vi "Teleop.vi"() -> ()   [LabVIEW 2017]
doc: "This VI is called for each TeleOp packet received from the DS where the robot is not disabled. It is often used to read from the joysticks and update I/O or to update setpoints for timed control loops. It should complete and return within 20 milliseconds or it may miss DS packets."
uses:
  <vilib>/Rock Robotics/WPI/DriverStation/WPI_DriverStationDerivedRobotMode.ctl
  <vilib>/Rock Robotics/WPI/DriverStation/WPI_DriverStationRobotMode2.ctl
  <vilib>/Rock Robotics/WPI/DriverStation/WPI_DriverStationMatch Info.ctl
  <vilib>/Rock Robotics/WPI/Joystick/WPI_JoystickDeviceEnum.ctl
  <vilib>/Rock Robotics/SystemInterfaces/DIO/FPGA_DIOPWMChannel.ctl
  <vilib>/Rock Robotics/SystemInterfaces/DIO/FPGA_DIOChannel.ctl
  <vilib>/Rock Robotics/WPI/MotorControl/WPI_MotorControlOpen SPARK.vi
  <vilib>/Rock Robotics/WPI/Switch/WPI_SwitchOpenLimit.vi
  <vilib>/Rock Robotics/WPI/RobotDrive/WPI_RobotDriveOpen2MotorWithSPARK.vi
  <vilib>/Rock Robotics/WPI/RobotDrive/WPI_RobotDriveArcadeDrive_Standard(NoSaturation).vi
panel:
  in  "Match Info":T1={"Autonomous Elapsed Seconds"=0.0, "TeleOp Elapsed Seconds"=0.0, "Disabled Elapsed Seconds"=0.0, "Visited Autonomous"=FALSE, "Visited TeleOp"=FALSE, "Visited Disabled"=FALSE, "Autonomous Settings"={"Autonomous Style"=enum."Independent", "VI Refnum"=refnum}}
  in  "Robot Mode":T2
  in  "Call Context":T3
  out "Switch Pressed 2":bool
  out "Switch Pressed":bool
  in  "stop 2":bool
  in  "stop":bool
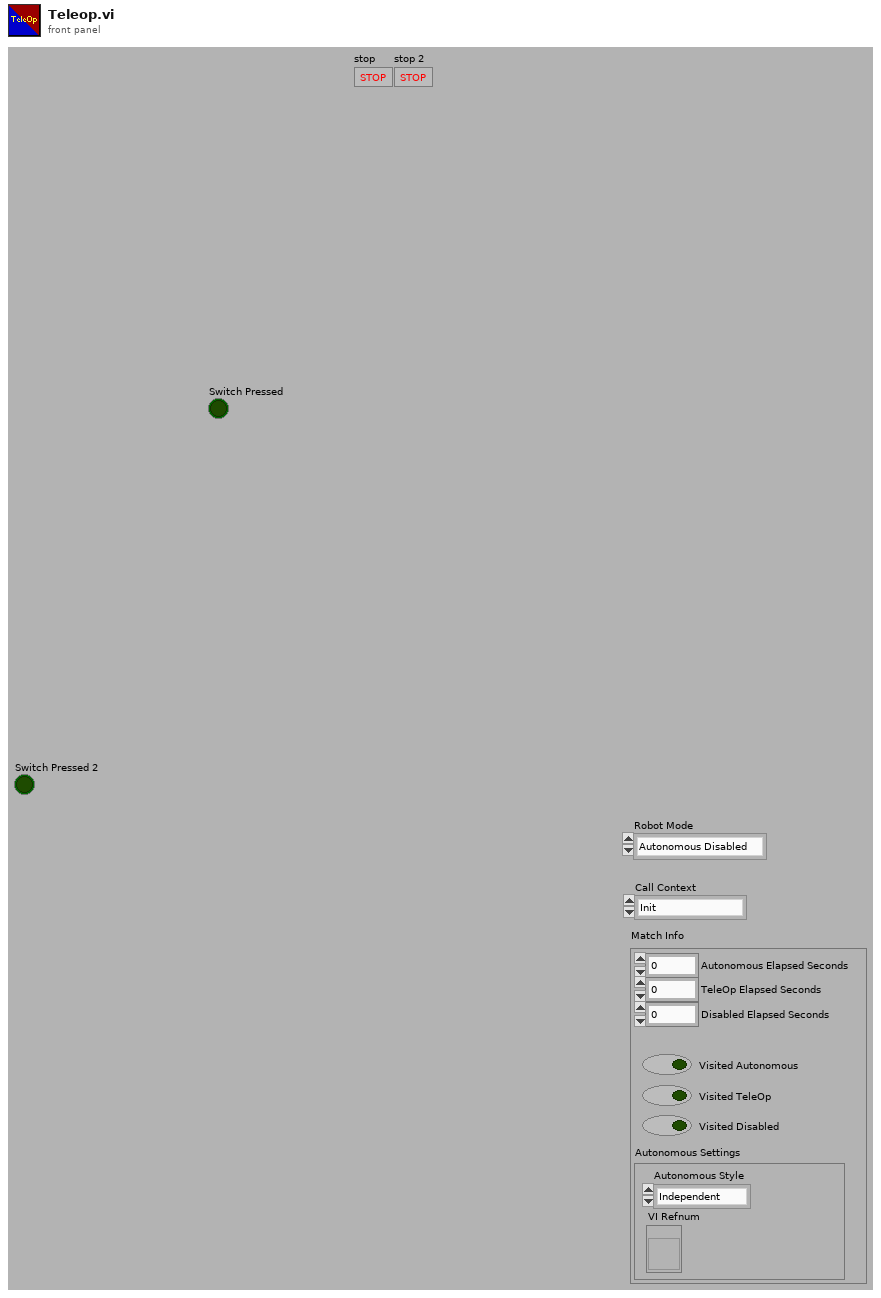
[diagram p1: front panel]
types:
  T1 = typedef "WPI_DriverStationMatch Info.ctl" = cluster{"Autonomous Elapsed Seconds":dbl, "TeleOp Elapsed Seconds":dbl, "Disabled Elapsed Seconds":dbl, "Visited Autonomous":bool, "Visited TeleOp":bool, "Visited Disabled":bool, "Autonomous Settings":cluster{"Autonomous Style":enum16{"Iterative", "Independent"}, "VI Refnum":refnum<vi>}}
  T2 = typedef "WPI_DriverStationRobotMode2.ctl" = enum16{"Autonomous Disabled", "Autonomous Enabled", "Teleop Disabled", "Teleop Enabled", "Disconnected", "Finish", "Test Disabled", "Test Enabled", "Emergency Stopped"}
  T3 = typedef "WPI_DriverStationDerivedRobotMode.ctl" = enum16{"Init", "Execute", "Stop"}
  T4 = typedef "FPGA_DIOPWMChannel.ctl" = enum8{"PWM 0", "PWM 1", "PWM 2", "PWM 3", "PWM 4", "PWM 5", "PWM 6", "PWM 7", "PWM 8", "PWM 9", "PWM MXP 0", "PWM MXP 1", "PWM MXP 2", "PWM MXP 3", "PWM MXP 4", "PWM MXP 5", "PWM MXP 6", "PWM MXP 7", "PWM MXP 8", "PWM MXP 9", "Invalid"}
  T5 = typedef "FPGA_DIOChannel.ctl" = enum8{"DIO 0", "DIO 1", "DIO 2", "DIO 3", "DIO 4", "DIO 5", "DIO 6", "DIO 7", "DIO 8", "DIO 9", "DIO MXP 0", "DIO MXP 1", "DIO MXP 2", "DIO MXP 3", "DIO MXP 4", "DIO MXP 5", "DIO MXP 6", "DIO MXP 7", "DIO MXP 8", "DIO MXP 9", "DIO MXP 10", "DIO MXP 11", "DIO MXP 12", "DIO MXP 13", "DIO MXP 14", "DIO MXP 15", "SPI Port CS1", "SPI Port CS2", "SPI Port CS3", "SPI Port MISO", "SPI Port MOSI", "Invalid"}
  T6 = typedef "WPI_JoystickDeviceEnum.ctl" = enum16{"USB 0", "USB 1", "USB 2", "USB 3", "USB 4", "USB 5"}
  T7 = typedef "WPI_MotorControlDeviceRef.ctl" = cluster{"DeviceStatus":errorcluster, "Type":T8, "PWM":cluster{"PWM Channel":T4, "DeadBand":T9}, "CAN":cluster{"Device Number":u8, "SetOutput VI Ref":variant, "GetOutput VI Ref":variant, "Enable VI Ref":variant, "Disable VI Ref":variant, "Data":variant}, "Invert":bool, "DIO PWM":cluster{"PWM \"Enable\" Channel":T4, "DIOChannel":T5, "PWM Rate":dbl}}
  T8 = typedef "WPI_MotorControlType.ctl" = enum16{"PWM", "CAN", "DIO PWM"}
  T9 = typedef "WPI_PWMDeadband.ctl" = cluster{"Name":string, "maxPositivePwm":i32, "minPositivePwm":i32, "centerPwm":i32, "maxNegativePwm":i32, "minNegativePwm":i32, "angularRange":u16}
  T10 = typedef "WPI_SwitchDevRef.ctl" = cluster{"DevStatus":errorcluster, "DIO Channel":T5, "CntIndex":T11, "Normally Closed":bool}
  T11 = typedef "FPGA_CounterCtrSystemIndex.ctl" = enum8{"Ctr 0", "Ctr 1", "Ctr 2", "Ctr 3", "Ctr 4", "Ctr 5", "Ctr 6", "Ctr 7", "Invalid"}
  T12 = typedef "WPI_JoystickDevRef.ctl" = cluster{"Device":T6}
  T13 = typedef "WPI_RobotDriveDevRef.ctl" = cluster{"DevStatus":errorcluster, "Motors[]":T7[], "Square Inputs":bool, "Max Output":dbl}
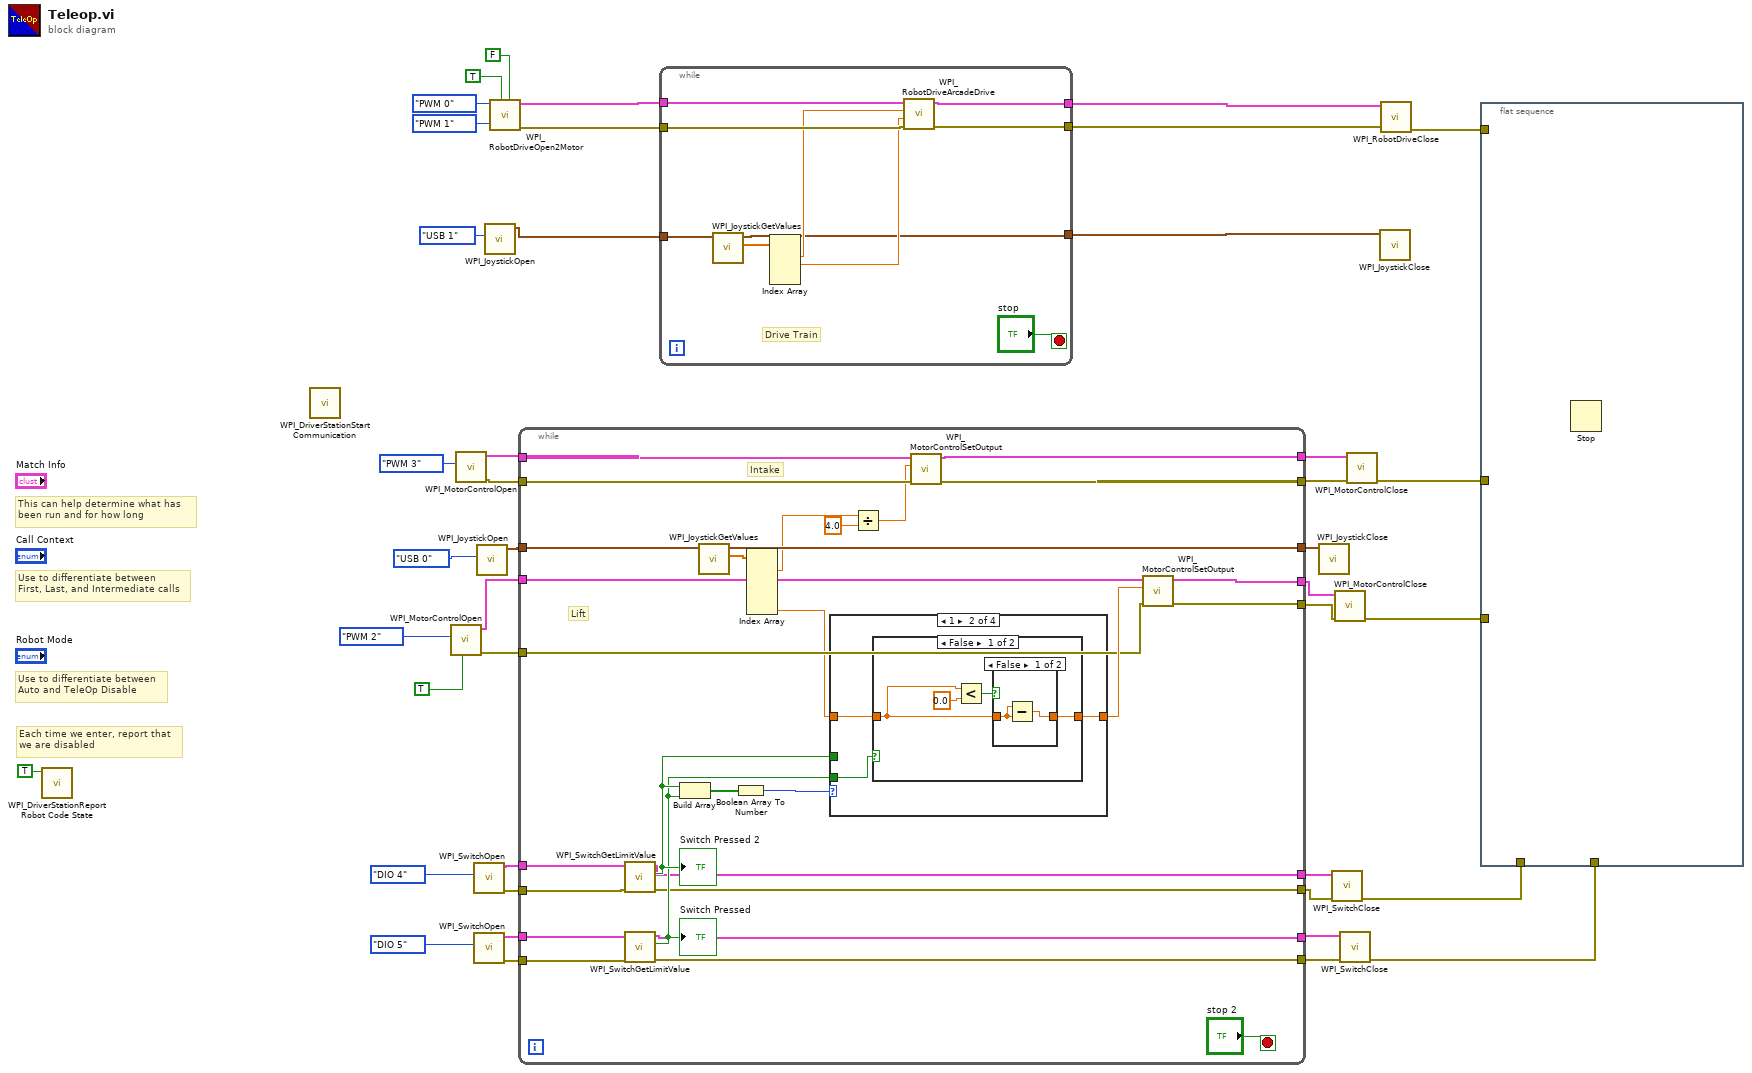
[diagram p0: block diagram]
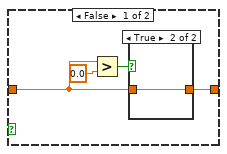
[diagram p6: hidden frame]
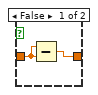
[diagram p7: hidden frame]
diagram:
  # "Each time we enter, report that\nwe are disabled"
  # "Use to differentiate between\nFirst, Last, and Intermediate calls"
  # "This can help determine what has\nbeen run and for how long"
  # "Use to differentiate between\nAuto and TeleOp Disable"
  n1 = call <vilib>:"WPI_DriverStationReport Robot Code State.vi"("Disabled"=TRUE ("Autonomous")) -> ()  [unwired: 10 in, 1 out]
  n2 = call <vilib>:"WPI_DriverStationStart Communication.vi"() -> ()  [unwired: 12 in]
  n3 = call-poly <vilib>:"WPI_MotorControlOpen.vi"("Invert"=TRUE, "PWM Channel"=FPGA_DIOPWMChannel."PWM 2" ("suck")) -> ("error out"=w15:errorcluster, "MotorControlDeviceRef"=w16:T7)  [unwired: 8 in]
  n4 = call-poly <vilib>:"WPI_MotorControlOpen.vi"("PWM Channel"=FPGA_DIOPWMChannel."PWM 3") -> ("error out"=w28:errorcluster, "MotorControlDeviceRef"=w31:T7)  [unwired: 9 in]
  n5 = call-poly <vilib>:"WPI_SwitchOpen.vi"("DIO Channel"=FPGA_DIOChannel."DIO 4") -> ("error out"=w19:errorcluster, "SwitchDevRef"=w20:T10)  [unwired: 9 in]
  n6 = call-poly <vilib>:"WPI_SwitchOpen.vi"("DIO Channel"=FPGA_DIOChannel."DIO 5") -> ("error out"=w17:errorcluster, "SwitchDevRef"=w18:T10)  [unwired: 9 in]
  n7 = call <vilib>:"WPI_JoystickOpen.vi"("JoystickDevice"=WPI_JoystickDeviceEnum."USB 0") -> ("JoystickDevRef"=w26:T12)  [unwired: 10 in]
  n8 = call <vilib>:"WPI_JoystickOpen.vi"("JoystickDevice"=WPI_JoystickDeviceEnum."USB 1") -> ("JoystickDevRef"=w41:T12)  [unwired: 10 in]
  n9 = call-poly <vilib>:"WPI_RobotDriveOpen2Motor.vi"("Right Motor Inverted"=FALSE, "Left Motor Inverted"=TRUE, "Right Motor"=FPGA_DIOPWMChannel."PWM 1", "Left Motor"=FPGA_DIOPWMChannel."PWM 0") -> ("error out"=w38:errorcluster, "RobotDriveDevRef"=w39:T13)  [unwired: 6 in]
  n10 = while {
    tunnel: w31 -> [w70]
    tunnel: [w69] -> w30
    tunnel: [w68] -> w29
    tunnel: w28 -> [w67]
    tunnel: w26 -> [w66]
    tunnel: [w64] -> w25
    tunnel: w20 -> [w58]
    tunnel: w19 -> [w57]
    tunnel: w18 -> [w56]
    tunnel: w17 -> [w55]
    tunnel: w16 -> [w54]
    tunnel: w15 -> [w53]
    tunnel: [w52] -> w9
    tunnel: [w51] -> w10
    tunnel: [w50] -> w14
    tunnel: [w49] -> w11
    tunnel: [w48] -> w12
    tunnel: [w47] -> w13
    stop <- "stop 2" stop-if-true
    # "Lift"
    # "Intake"
    n11 = call <vilib>:"WPI_SwitchGetLimitValue.vi"("error in (no error)"=w57, "SwitchDevRef"=w58) -> ("error out"=w49:errorcluster, "Switch Pressed"=w60:bool, "SwitchDevRef"=w50:T10)  [unwired: 7 in]
    "Switch Pressed 2" <- w60
    n12 = call <vilib>:"WPI_SwitchGetLimitValue.vi"("error in (no error)"=w55, "SwitchDevRef"=w56) -> ("error out"=w47:errorcluster, "Switch Pressed"=w59:bool, "SwitchDevRef"=w48:T10)  [unwired: 7 in]
    "Switch Pressed" <- w59
    n13 = Build Array(w60, w59) -> (w63:bool[])
    n14 = call <vilib>:"WPI_JoystickGetValues.vi"("JoystickDevRef"=w66) -> ("Axes"=w65:dbl[], "JoystickDevRef"=w64:T12)  [unwired: 6 in, 3 out]
    n15 = Boolean Array To Number(Boolean array=w63) -> (number=w62:u32)
    n16 = Index Array(array=w65) -> (element #1=w43:dbl, element #6=w42:dbl)  [unwired: 6 in, 4 out]
    n17 = case shown="1" w62 {
      tunnel: [w71 w74 w85 w94] -> w61
      tunnel: w59 -> [_ w73 _ _]
      tunnel: w60 -> [_ _ w84 _]
      tunnel: w42 -> [w71 w72 w83 w94]
      frame 0, Default {
      }
      frame 1 {
        n18 = case shown="False" w73 {
          tunnel: [w76 w82] -> w74
          tunnel: w72 -> [w75 w82]
          frame False {
            n19 = Less?(x=w75, y=0.0) -> (x < y?=w77:bool)
            n20 = case shown="False" w77 {
              tunnel: [w80 w81] -> w76
              tunnel: w75 -> [w79 w81]
              frame False {
                n21 = Subtract(x=w79, y=w79) -> (x-y=w80:dbl)
              }
              frame True {
              }
            }
          }
          frame True {
          }
        }
      }
      frame 2 {
        n22 = case shown="True" w84 {
          tunnel: [w87 w93] -> w85
          tunnel: w83 -> [w86 w93]
          frame False {
            n23 = Greater?(x=w86, y=0.0) -> (0:w88:bool)
            n24 = case shown="True" w88 {
              tunnel: [w91 w92] -> w87
              tunnel: w86 -> [w90 w92]
              frame False {
                n25 = Subtract(x=w90, y=w90) -> (x-y=w91:dbl)
              }
              frame True {
              }
            }
          }
          frame True {
          }
        }
      }
      frame 3 {
      }
    }
    n26 = Divide(x=w43, y=4.0) -> (x/y=w45:dbl)
    n27 = call <vilib>:"WPI_MotorControlSetOutput.vi"("error in (no error)"=w67, "Output"=w45, "MotorControlDevRef"=w70) -> ("error out"=w68:errorcluster, "MotorControlDevRef"=w69:T7)  [unwired: 6 in, 1 out]
    n28 = call <vilib>:"WPI_MotorControlSetOutput.vi"("error in (no error)"=w53, "Output"=w61, "MotorControlDevRef"=w54) -> ("error out"=w52:errorcluster, "MotorControlDevRef"=w51:T7)  [unwired: 6 in, 1 out]
  }
  n29 = while {
    tunnel: w41 -> [w103]
    tunnel: w39 -> [w102]
    tunnel: w38 -> [w101]
    tunnel: [w97] -> w35
    tunnel: [w96] -> w34
    tunnel: [w95] -> w33
    stop <- "stop" stop-if-true
    # "Drive Train"
    n30 = call <vilib>:"WPI_JoystickGetValues.vi"("JoystickDevRef"=w103) -> ("Axes"=w100:dbl[], "JoystickDevRef"=w95:T12)  [unwired: 6 in, 3 out]
    n31 = Index Array(array=w100) -> (element #1=w99:dbl, element #2=w98:dbl)  [unwired: 4 in, 2 out]
    n32 = call-poly <vilib>:"WPI_RobotDriveArcadeDrive.vi"("error in (no error)"=w101, "Y axis value"=w98, "X axis value"=w99, "RobotDriveDevRef"=w102) -> ("error out"=w96:errorcluster, "RobotDriveDevRef"=w97:T13)  [unwired: 5 in, 1 out]
  }
  n33 = call <vilib>:"WPI_JoystickClose.vi"("JoystickDevRef"=w25) -> ()  [unwired: 11 in]
  n34 = call <vilib>:"WPI_SwitchClose.vi"("error in (no error)"=w11, "SwitchDevRef"=w14) -> ("error out"=w6:errorcluster)  [unwired: 9 in]
  n35 = call <vilib>:"WPI_MotorControlClose.vi"("error in"=w9, "MotorControlDevRef"=w10) -> ("error out"=w2:errorcluster)  [unwired: 9 in]
  n36 = call <vilib>:"WPI_SwitchClose.vi"("error in (no error)"=w13, "SwitchDevRef"=w12) -> ("error out"=w5:errorcluster)  [unwired: 9 in]
  n37 = call <vilib>:"WPI_MotorControlClose.vi"("error in"=w29, "MotorControlDevRef"=w30) -> ("error out"=w3:errorcluster)  [unwired: 9 in]
  n38 = call <vilib>:"WPI_JoystickClose.vi"("JoystickDevRef"=w33) -> ()  [unwired: 11 in]
  n39 = call <vilib>:"WPI_RobotDriveClose.vi"("error in (no error)"=w34, "RobotDriveDevRef"=w35) -> ("error out"=w4:errorcluster)  [unwired: 9 in]
  n40 = flat-sequence {
    tunnel: w6 -> [_]
    tunnel: w5 -> [_]
    tunnel: w4 -> [_]
    tunnel: w3 -> [_]
    tunnel: w2 -> [_]
    frame #0 {
      n41 = Stop() -> ()  [unwired: 1 in]
    }
  }
